vi "读取能否飞行.vi"(8 "error in (no error)":errorcluster caption="错误输入（无错误）", 11 "Animal输入":refnum<class "Animal.lvclass">) -> (0 "error out":errorcluster caption="错误输出", 2 "能否飞行":bool, 3 "Animal输出":refnum<class "Animal.lvclass">)   [LabVIEW 2020, in "Animal.lvclass"]
uses:
  Animal.lvclass
  Animal.lvclass/Animal.ctl
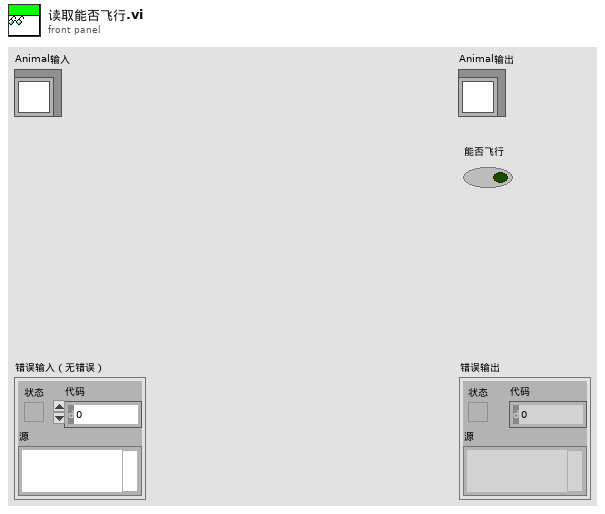
[diagram p1: front panel]
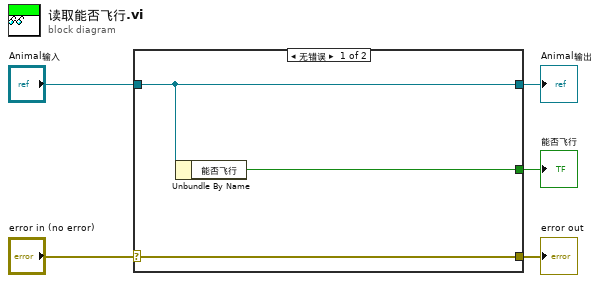
[diagram p0: block diagram]
diagram:
  n1 = case shown="无错误" "error in (no error)" {
    selector: "error in (no error)" -> [w8 w9]
    tunnel: [w8 w9] -> w4
    tunnel: [w7 w10] -> w2
    tunnel: "Animal输入" -> [w7 w10]
    tunnel: [w6 _] -> w1
    frame No Error {
      n2 = Unbundle By Name(w7) -> ("能否飞行"=w6:bool)
    }
    frame Error {
    }
  }
  "error out" <- w4
  "Animal输出" <- w2
  "能否飞行" <- w1
